vi "SPD.Save2DArray.vi"(8 "Error In":errorcluster, 10 "Array":dbl[][](array[numeric]), 11 "File Path":path) -> (0 "Error Out":errorcluster)   [LabVIEW 2018]
uses:
  <vilib>/Utility/file.llb/Write Delimited Spreadsheet (DBL).vi
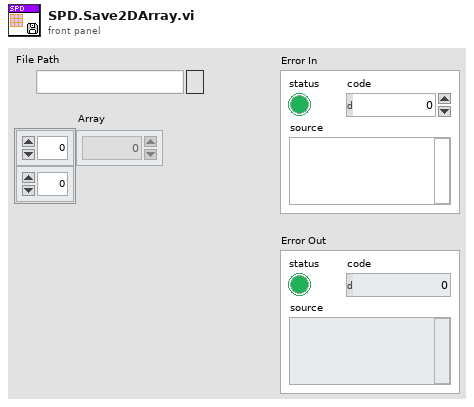
[diagram p1: front panel]
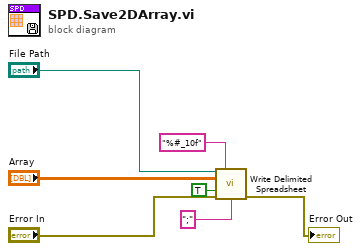
[diagram p0: block diagram]
diagram:
  n1 = call-poly <vilib>:"Write Delimited Spreadsheet.vi"("file path (dialog if empty)"="File Path", "format (%.3f)"="%#_10f", "2D data"="Array", "append to file? (new file:F)"=TRUE, "error in (no error)"="Error In", "delimiter (\\t)"=";" ("delimiter (\\t)")) -> ("error out"=→"Error Out":errorcluster)  [unwired: 8 in, 1 out]
